vi "FTW-ZMQ-Context-Destroy.vi"(0 "ZeroMQ Context":refnum<class "FTW-ZMQ-Context.lvclass">, 5 "Force Destroy all open Sockets?":bool, 11 "error in":errorcluster) -> (15 "error out":errorcluster)   [LabVIEW 2014, in "FTW-ZMQ-Context.lvclass"]
uses:
  FTW-ZMQ-Context.lvclass
  FTW-ZMQ-Context.lvclass/FTW-ZMQ-Context.ctl
panel:
  # "Inputs"
  # "Outputs"
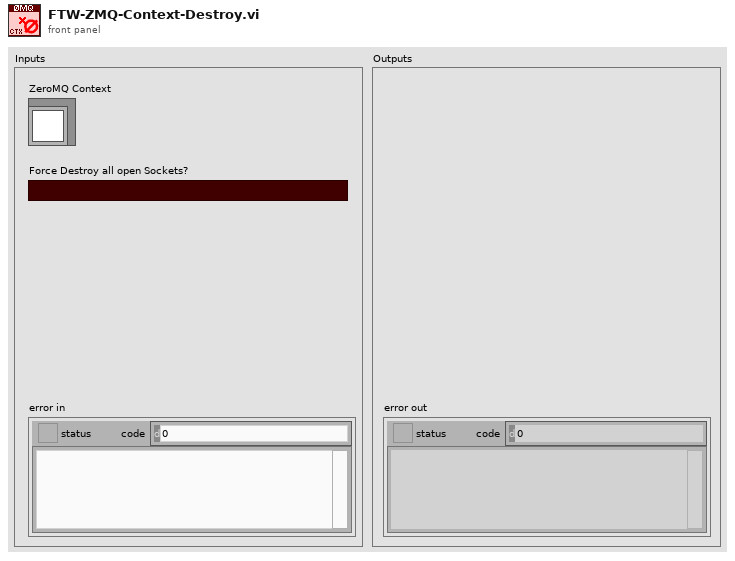
[diagram p1: front panel]
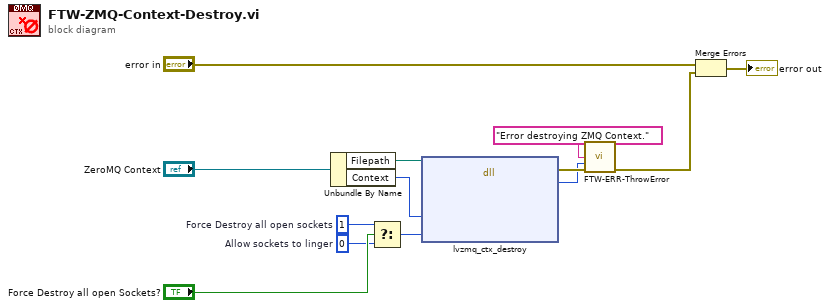
[diagram p0: block diagram]
diagram:
  w3 = 1  # Force Destroy all open sockets
  w1 = 0  # Allow sockets to linger
  n1 = Unbundle By Name("ZeroMQ Context") -> ("Filepath"=w12:path, "Context"=w11:u64)
  n2 = Select(t=w3, s="Force Destroy all open Sockets?", f=w1) -> (s? t:f=w2:i32)
  n3 = dll-call lib="?" fn="lvzmq_ctx_destroy" ("zmq_labview.dll:lvzmq_term")(path in=w12, "Context"=w11, "Flags"=w2) -> (error out=w9:errorcluster, "Return Value"=w8:i32)  [unwired: 6 in, 1 out]
  n4 = call "FTW-ERR-ThrowError.vi"("Error Message"="Error destroying ZMQ Context.", "Error Code"=w8, "error in"=w9) -> ("error out"=w6:errorcluster)  [unwired: 12 in]
  n5 = Merge Errors("error in", w6) -> (→"error out":errorcluster)
